vi "After Launch Init.vi"(8 "error in (no error)":errorcluster, 11 "Camera Actor in":refnum<class "Camera Actor.lvclass">) -> (0 "error out":errorcluster, 3 "Camera Actor out":refnum<class "Camera Actor.lvclass">)   [LabVIEW 2020, in "Camera Actor.lvlib" / "Camera Actor.lvclass"]
uses:
  Camera Actor.lvclass
  Camera Actor.lvclass/Camera Actor.ctl
  Logbook/Logbook/Logbook.lvclass
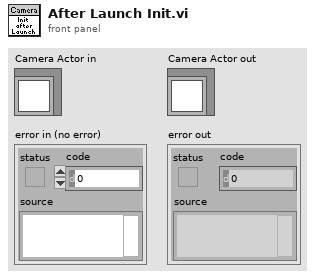
[diagram p1: front panel]
types:
  T1 = typedef "Image Type" = u32
  T2 = typedef "IMAQ Image.ctl" = refnum<image>
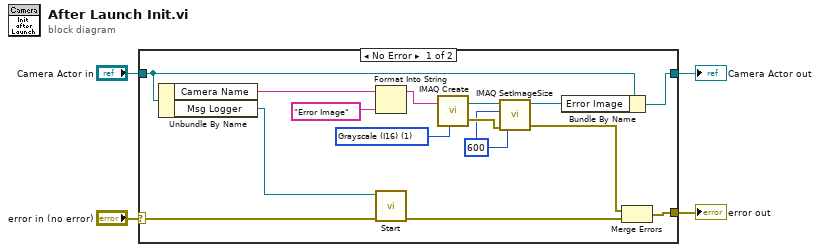
[diagram p0: block diagram]
diagram:
  n1 = case shown="No Error" "error in (no error)" {
    selector: "error in (no error)" -> [w18 w21]
    tunnel: [w10 w21] -> w3
    tunnel: [w16 w20] -> w1
    tunnel: "Camera Actor in" -> [w15 w20]
    frame No Error {
      w5 = 600 ("Y Resolution")
      w9 = T1 1 items=["Grayscale (U8)", "Grayscale (I16)", "Grayscale (SGL)", "Complex (CSG)", "RGB (U32)", "HSL (U32)", "RGB (U64)", "Grayscale (U16)"] ("Image Type")
      n2 = Unbundle By Name(w15) -> ("Camera Name"=w14:string, "Msg Logger"=w19:refnum<class "Logbook.lvclass">)
      n3 = Format Into String(initial string=w14, "Error Image" ("Camera Name")) -> (resulting string=w13:string)  [unwired: 2 in, 1 out]
      n4 = call-dynamic "Start.vi"("error in (no error)"=w18, "Logbook in"=w19) -> ("error out"=w17:errorcluster)  [unwired: 8 in, 1 out]
      n5 = call "IMAQ Create"("Image Name"=w13, "Image Type"=w9) -> ("New Image"=w11:T2, "error out"=w7:errorcluster)  [unwired: 3 in]
      n6 = call "IMAQ SetImageSize"("error in (no error)"=w7, "Y Resolution"=w5, "X Resolution"=w5, "Image"=w11) -> ("error out"=w6:errorcluster, "Image Out"=w8:T2)  [unwired: 1 in]
      n7 = Bundle By Name(cluster=w15, "Error Image"=w8) -> (w16:refnum<class "Camera Actor.lvclass">)
      n8 = Merge Errors(w6, w17) -> (w10:errorcluster)
    }
    frame Error {
    }
  }
  "error out" <- w3
  "Camera Actor out" <- w1
